vi "Compute Guess Fit Parameters.vi"(8 "error in (no error)":errorcluster, 9 "Additional Data":variant, 10 "Fit Model":T2, 11 "Data in":T3) -> (0 "error out":errorcluster, 1 "Additional LM Data":variant, 3 "Initial Fit Parameters":dbl[](array[numeric]), 4 "Parameter Bounds":T1={"parameter minimum"=[0.0, -inf, 0.0], "parameter maximum"=[inf, inf, inf]})   [LabVIEW 2019]
uses:
  Fit Models.ctl
  N Components Additional Fit Settings.ctl
  D-Only Fixed Parameters.ctl
  <vilib>/Utility/error.llb/DialogType.ctl
  <vilib>/Analysis/NI_AALPro.lvlib
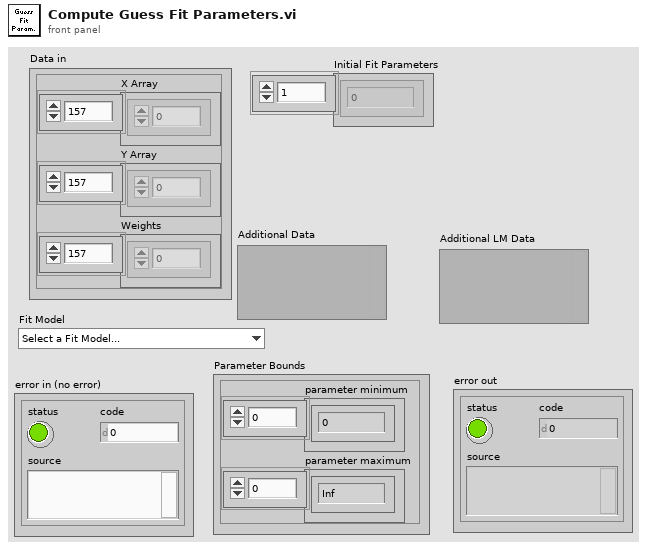
[diagram p1: front panel]
types:
  T1 = cluster{"parameter minimum":dbl[], "parameter maximum":dbl[]}
  T2 = typedef "Fit Models.ctl" = enum16{"Select a Fit Model...", "           Single Peak", "Gaussian", "Asymmetric Gaussian", "Lorentzian", "Asymmetric Lorentzian", "Gaussian/Lorentzian", "Lorentzian/Gaussian", "           Double Peak", "Two Gaussians", "Two Asymmetric Gaussians", "Two H-Connected Gaussians", "Two T-Connected Gaussians", "Two H-Connected Asymmetric Gaussians", "Two T-Connected Asymmetric Gaussians", "           Triple Peak", "Three Gaussians", "Three Asymmetric Gaussians", "              Decays", "Single Exponential", "Two Exponentials", "               ACF", "2D Gaussian ACF", "2D Gaussian + Blinking ACF", "2D Gaussian + Flow ACF", "3D Gaussian ACF", "3D Gaussian + Blinking ACF", "             Multiplot", "2D Gaussian ACF & 2D Gaussian + Flow ACF"}
  T3 = cluster{"X Array":dbl[], "Y Array":dbl[], "Weights":dbl[]}
  T4 = typedef "N Components Additional Fit Settings.ctl" = cluster{"Fixed Parameters":T5, "Cursor Coordinates":dbl[], "Data Split Point":i32}
  T5 = typedef "D-Only Fixed Parameters.ctl" = cluster{"Fix D-only Peak Location":bool, "Peak Location":dbl, "Fix D-only Peak FWHM":bool, "Peak FWHM":dbl}
  T6 = cluster{"initial amplitude":dbl, "initial center":dbl, "initial standard deviation":dbl, "offset":dbl}
  T7 = cluster{"amp min":dbl, "amp max":dbl, "damping min":dbl, "damping max":dbl, "offset min":dbl, "offset max":dbl}
  T8 = typedef "DialogType.ctl" = u16
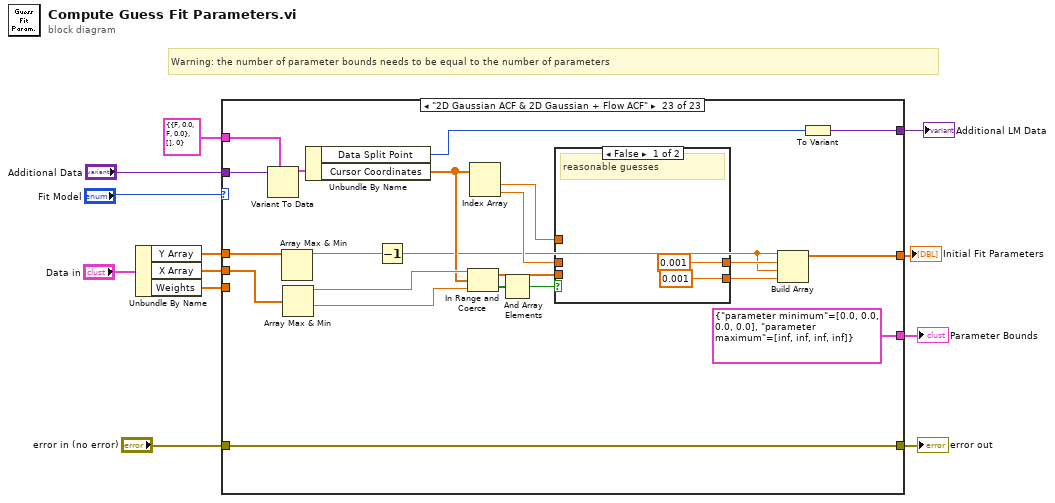
[diagram p0: block diagram]
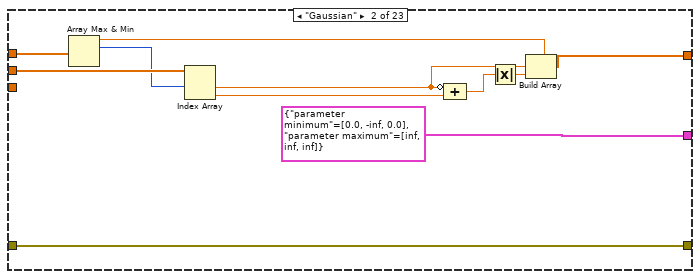
[diagram p3: hidden frame]
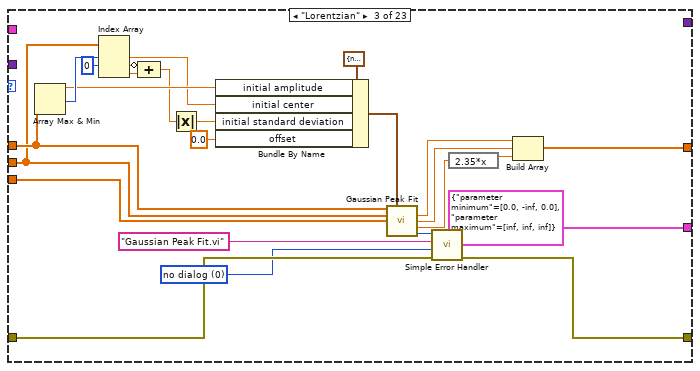
[diagram p4: hidden frame]
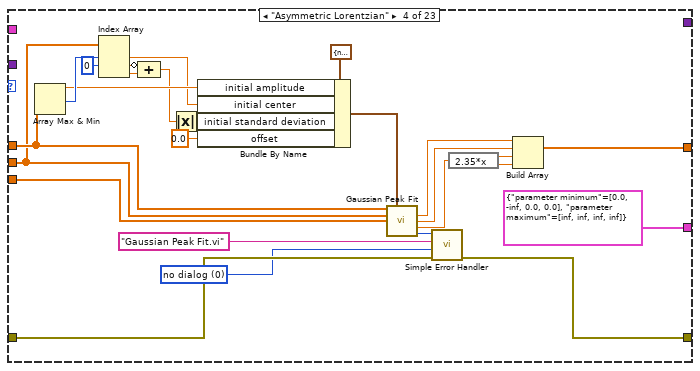
[diagram p5: hidden frame]
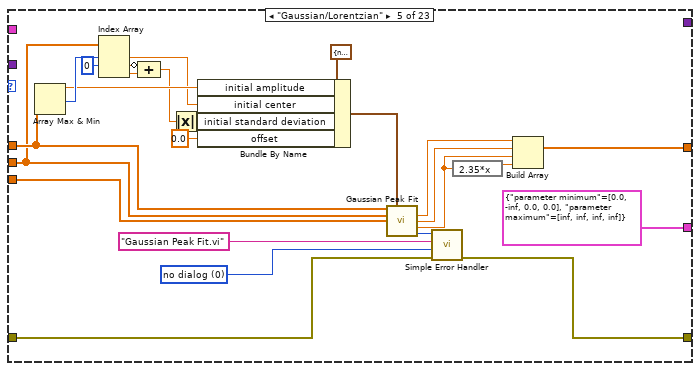
[diagram p6: hidden frame]
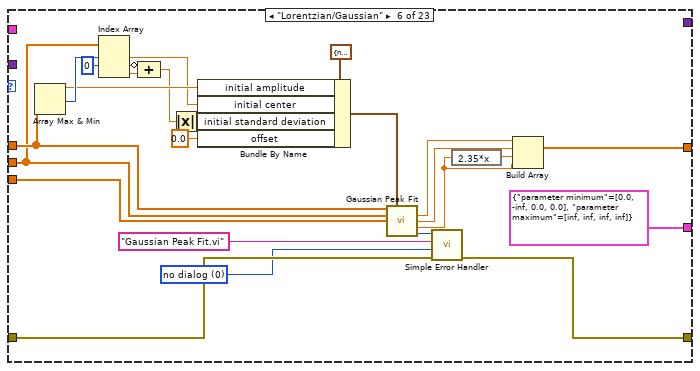
[diagram p7: hidden frame]
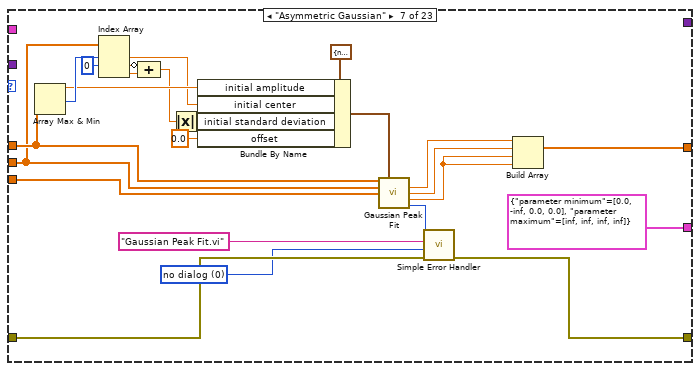
[diagram p8: hidden frame]
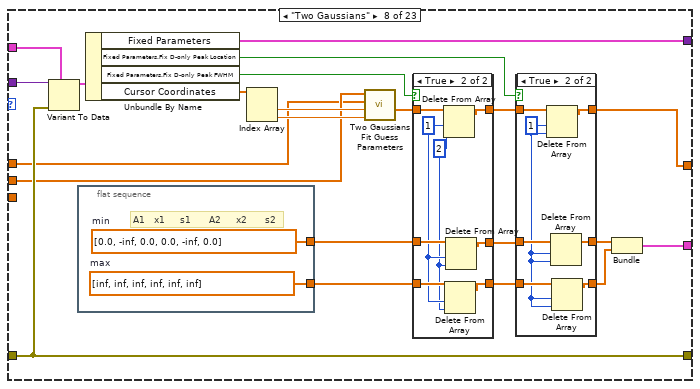
[diagram p9: hidden frame]
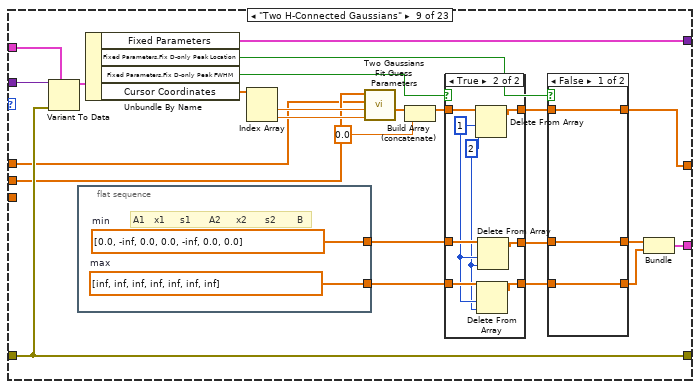
[diagram p12: hidden frame]
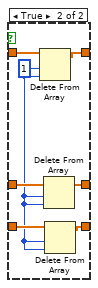
[diagram p14: hidden frame]
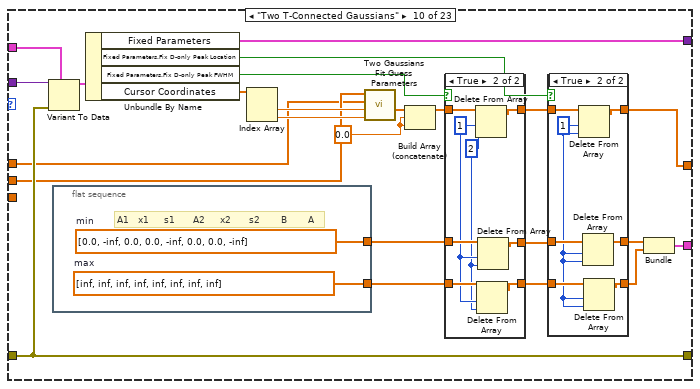
[diagram p15: hidden frame]
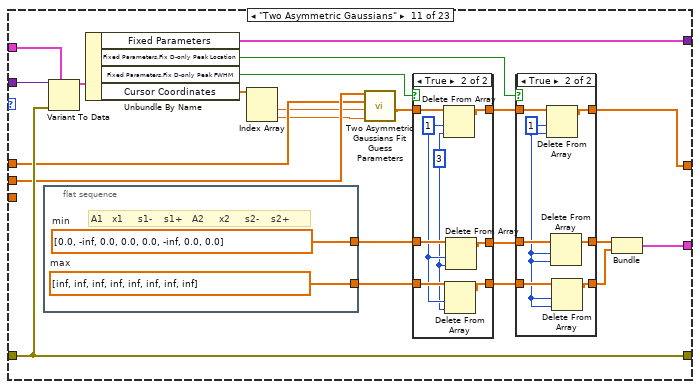
[diagram p18: hidden frame]
diagram:
  # "Warning: the number of parameter bounds needs to be equal to the number of parameters"
  n1 = Unbundle By Name("Data in") -> ("Y Array"=w8:dbl[], "X Array"=w7:dbl[], "Weights"=w6:dbl[])
  n2 = case shown="\"2D Gaussian ACF & 2D Gaussian + Flow ACF\"" "Fit Model" {
    tunnel: "error in (no error)" -> [w13 w24 w49 w74 w99 w124 w148 w169 w216 w263 w308 w355 w402 w446 w492 w523 w535 w552 w576 w601 w623 w648 w674]
    tunnel: [_ w15 w45 w71 w97 w122 w146 w154 w201 w248 w298 w335 w382 w437 w480 w518 w532 w549 w573 w598 w620 w645 w671] -> w11
    tunnel: [w13 w24 w43 w69 w95 w120 w144 w169 w216 w263 w308 w355 w402 w446 w492 w523 w535 w552 w576 w601 w623 w648 w674] -> w10
    tunnel: w8 -> [_ w22 w32 w58 w84 w109 w133 w163 w210 w257 w292 w339 w386 w431 w489 w526 w534 w551 w575 w600 w622 w647 w673]
    tunnel: w7 -> [_ w23 w31 w57 w83 w108 w132 w164 w211 w258 w293 w340 w387 w432 w490 w527 w533 w539 w564 w589 w609 w636 w663]
    tunnel: w6 -> [_ _ w39 w65 w91 w116 w140 _ _ _ _ _ _ _ _ w525 _ _ _ _ _ _ _]
    tunnel: [_ T1 {"parameter minimum"=[0.0, -inf, 0.0], "parameter maximum"=[inf, inf, inf]} ("Parameter Bounds") T1 {"parameter minimum"=[0.0, -inf, 0.0], "parameter maximum"=[inf, inf, inf]} ("Parameter Bounds") T1 {"parameter minimum"=[0.0, -inf, 0.0, 0.0], "parameter maximum"=[inf, inf, inf, inf]} ("Parameter Bounds") T1 {"parameter minimum"=[0.0, -inf, 0.0, 0.0], "parameter maximum"=[inf, inf, inf, inf]} ("Parameter Bounds") T1 {"parameter minimum"=[0.0, -inf, 0.0, 0.0], "parameter maximum"=[inf, inf, inf, inf]} ("Parameter Bounds") T1 {"parameter minimum"=[0.0, -inf, 0.0, 0.0], "parameter maximum"=[inf, inf, inf, inf]} ("Parameter Bounds") w151 w198 w245 w295 w342 w389 w434 w477 T1 {"parameter minimum"=[0.0, 0.0], "parameter maximum"=[inf, inf]} ("parameter bounds") T1 {"parameter minimum"=[0.0, 0.0, 0.0, 0.0], "parameter maximum"=[inf, inf, inf, inf]} ("parameter bounds") T1 {"parameter minimum"=[0.0, 0.0], "parameter maximum"=[inf, inf]} ("Parameter Bounds") T1 {"parameter minimum"=[0.0, 0.0, 0.0, 0.0], "parameter maximum"=[inf, inf, inf, inf]} ("Parameter Bounds") T1 {"parameter minimum"=[0.0, 0.0, 0.0], "parameter maximum"=[inf, inf, inf]} ("Parameter Bounds") T1 {"parameter minimum"=[0.0, 0.0, 0.0], "parameter maximum"=[inf, inf, inf]} ("Parameter Bounds") T1 {"parameter minimum"=[0.0, 0.0, 0.0, 0.0, 0.0], "parameter maximum"=[inf, inf, inf, inf, inf]} ("Parameter Bounds") T1 {"parameter minimum"=[0.0, 0.0, 0.0, 0.0], "parameter maximum"=[inf, inf, inf, inf]} ("Parameter Bounds")] -> w4
    tunnel: "Additional Data" -> [_ _ _ _ _ _ _ w170 w217 w264 w309 w356 w403 w447 w493 _ _ w547 w571 w596 w618 w643 w669]
    tunnel: [_ _ _ _ _ _ _ w150 w197 w244 w294 w341 w388 w433 w476 _ _ _ _ _ _ _ w653] -> w2
    tunnel: T4 {"Fixed Parameters"={"Fix D-only Peak Location"=FALSE, "Peak Location"=0.0, "Fix D-only Peak FWHM"=FALSE, "Peak FWHM"=0.0}, "Cursor Coordinates"=[], "Data Split Point"=0} ("N Components Additional Fit Settings") -> [_ _ _ _ _ _ _ w149 w194 w241 w288 w333 w380 w427 w473 _ _ w536 w555 w582 w606 w626 w657]
    frame "Select a Fit Model...", Default {
    }
    frame "Gaussian" {
      n3 = Array Max & Min(array=w22) -> (max value=w20:dbl, max index (indices)=w21:i32)  [unwired: 2 out]
      n4 = Index Array(array=w23, index #1=w21) -> (element #1=w19:dbl, element #2=w18:dbl)  [unwired: 1 in]
      n5 = Compound Arithmetic op=ADD(invert w19, w18) -> (w17:dbl)
      n6 = Absolute Value(x=w17) -> (abs(x)=w16:dbl)
      n7 = Build Array(w20, w19, w16) -> (w15:dbl[])
    }
    frame "Lorentzian" {
      w42 = T8 0 items=["no dialog", "OK message", "continue or stop message", "OK message + warnings", "continue/stop + warnings"] ("type of dialog (OK msg:1)")
      n8 = Array Max & Min(array=w32) -> (max value=w35:dbl, max index (indices)=w37:i32)  [unwired: 2 out]
      n9 = Index Array(array=w31, index #1=w37, index #2=0 ("index")) -> (element #1=w34:dbl, element #2=w29:dbl, element #3=w28:dbl)  [unwired: 1 in]
      n10 = Compound Arithmetic op=ADD(invert w29, w28) -> (w27:dbl)
      n11 = Absolute Value(x=w27) -> (abs(x)=w26:dbl)
      n12 = Bundle By Name(cluster=T6 {"initial amplitude"=nan, "initial center"=nan, "initial standard deviation"=nan, "offset"=nan} ("initial guess"), "initial amplitude"=w35, "initial center"=w34, "initial standard deviation"=w26, "offset"=0.0) -> (w25:T6)
      n13 = call <vilib>:"Gaussian Peak Fit.vi"("Y"=w32, "initial guess"=w25, "X"=w31, "Weight"=w39) -> ("amplitude"=w44:dbl, "center"=w46:dbl, "standard deviation"=w47:dbl, "error"=w41:i32)  [unwired: 5 in, 3 out]
      n14 = call <vilib>:"Simple Error Handler.vi"("error code (no error:0)"=w41, "error source (\" \")"="Gaussian Peak Fit.vi" ("error source (\" \")"), "type of dialog (OK msg:1)"=w42, "error in (no error)"=w49) -> ("error out"=w43:errorcluster)  [unwired: 1 in, 4 out]
      n15 = expression code="2.35*x"(w47) -> (w48:dbl)
      n16 = Build Array(w44, w46, w48) -> (w45:dbl[])
    }
    frame "Asymmetric Lorentzian" {
      w68 = T8 0 items=["no dialog", "OK message", "continue or stop message", "OK message + warnings", "continue/stop + warnings"] ("type of dialog (OK msg:1)")
      n17 = Array Max & Min(array=w58) -> (max value=w61:dbl, max index (indices)=w63:i32)  [unwired: 2 out]
      n18 = Index Array(array=w57, index #1=w63, index #2=0 ("index")) -> (element #1=w60:dbl, element #2=w55:dbl, element #3=w54:dbl)  [unwired: 1 in]
      n19 = Compound Arithmetic op=ADD(invert w55, w54) -> (w53:dbl)
      n20 = Absolute Value(x=w53) -> (abs(x)=w52:dbl)
      n21 = Bundle By Name(cluster=T6 {"initial amplitude"=nan, "initial center"=nan, "initial standard deviation"=nan, "offset"=nan} ("initial guess"), "initial amplitude"=w61, "initial center"=w60, "initial standard deviation"=w52, "offset"=0.0) -> (w51:T6)
      n22 = call <vilib>:"Gaussian Peak Fit.vi"("Y"=w58, "initial guess"=w51, "X"=w57, "Weight"=w65) -> ("amplitude"=w70:dbl, "center"=w72:dbl, "standard deviation"=w73:dbl, "error"=w67:i32)  [unwired: 5 in, 3 out]
      n23 = call <vilib>:"Simple Error Handler.vi"("error code (no error:0)"=w67, "error source (\" \")"="Gaussian Peak Fit.vi" ("error source (\" \")"), "type of dialog (OK msg:1)"=w68, "error in (no error)"=w74) -> ("error out"=w69:errorcluster)  [unwired: 1 in, 4 out]
      n24 = expression code="2.35*x"(w73) -> (w50:dbl)
      n25 = Build Array(w70, w72, w50, w50) -> (w71:dbl[])
    }
    frame "Gaussian/Lorentzian" {
      w94 = T8 0 items=["no dialog", "OK message", "continue or stop message", "OK message + warnings", "continue/stop + warnings"] ("type of dialog (OK msg:1)")
      n26 = Array Max & Min(array=w84) -> (max value=w87:dbl, max index (indices)=w89:i32)  [unwired: 2 out]
      n27 = Index Array(array=w83, index #1=w89, index #2=0 ("index")) -> (element #1=w86:dbl, element #2=w81:dbl, element #3=w80:dbl)  [unwired: 1 in]
      n28 = Compound Arithmetic op=ADD(invert w81, w80) -> (w79:dbl)
      n29 = Absolute Value(x=w79) -> (abs(x)=w78:dbl)
      n30 = Bundle By Name(cluster=T6 {"initial amplitude"=nan, "initial center"=nan, "initial standard deviation"=nan, "offset"=nan} ("initial guess"), "initial amplitude"=w87, "initial center"=w86, "initial standard deviation"=w78, "offset"=0.0) -> (w77:T6)
      n31 = call <vilib>:"Gaussian Peak Fit.vi"("Y"=w84, "initial guess"=w77, "X"=w83, "Weight"=w91) -> ("amplitude"=w96:dbl, "center"=w98:dbl, "standard deviation"=w75:dbl, "error"=w93:i32)  [unwired: 5 in, 3 out]
      n32 = call <vilib>:"Simple Error Handler.vi"("error code (no error:0)"=w93, "error source (\" \")"="Gaussian Peak Fit.vi" ("error source (\" \")"), "type of dialog (OK msg:1)"=w94, "error in (no error)"=w99) -> ("error out"=w95:errorcluster)  [unwired: 1 in, 4 out]
      n33 = expression code="2.35*x"(w75) -> (w76:dbl)
      n34 = Build Array(w96, w98, w75, w76) -> (w97:dbl[])
    }
    frame "Lorentzian/Gaussian" {
      w119 = T8 0 items=["no dialog", "OK message", "continue or stop message", "OK message + warnings", "continue/stop + warnings"] ("type of dialog (OK msg:1)")
      n35 = Array Max & Min(array=w109) -> (max value=w112:dbl, max index (indices)=w114:i32)  [unwired: 2 out]
      n36 = Index Array(array=w108, index #1=w114, index #2=0 ("index")) -> (element #1=w111:dbl, element #2=w106:dbl, element #3=w105:dbl)  [unwired: 1 in]
      n37 = Compound Arithmetic op=ADD(invert w106, w105) -> (w104:dbl)
      n38 = Absolute Value(x=w104) -> (abs(x)=w103:dbl)
      n39 = Bundle By Name(cluster=T6 {"initial amplitude"=nan, "initial center"=nan, "initial standard deviation"=nan, "offset"=nan} ("initial guess"), "initial amplitude"=w112, "initial center"=w111, "initial standard deviation"=w103, "offset"=0.0) -> (w102:T6)
      n40 = call <vilib>:"Gaussian Peak Fit.vi"("Y"=w109, "initial guess"=w102, "X"=w108, "Weight"=w116) -> ("amplitude"=w121:dbl, "center"=w123:dbl, "standard deviation"=w100:dbl, "error"=w118:i32)  [unwired: 5 in, 3 out]
      n41 = call <vilib>:"Simple Error Handler.vi"("error code (no error:0)"=w118, "error source (\" \")"="Gaussian Peak Fit.vi" ("error source (\" \")"), "type of dialog (OK msg:1)"=w119, "error in (no error)"=w124) -> ("error out"=w120:errorcluster)  [unwired: 1 in, 4 out]
      n42 = expression code="2.35*x"(w100) -> (w101:dbl)
      n43 = Build Array(w121, w123, w101, w100) -> (w122:dbl[])
    }
    frame "Asymmetric Gaussian" {
      w143 = T8 0 items=["no dialog", "OK message", "continue or stop message", "OK message + warnings", "continue/stop + warnings"] ("type of dialog (OK msg:1)")
      n44 = Array Max & Min(array=w133) -> (max value=w136:dbl, max index (indices)=w138:i32)  [unwired: 2 out]
      n45 = Index Array(array=w132, index #1=w138, index #2=0 ("index")) -> (element #1=w135:dbl, element #2=w130:dbl, element #3=w129:dbl)  [unwired: 1 in]
      n46 = Compound Arithmetic op=ADD(invert w130, w129) -> (w128:dbl)
      n47 = Absolute Value(x=w128) -> (abs(x)=w127:dbl)
      n48 = Bundle By Name(cluster=T6 {"initial amplitude"=nan, "initial center"=nan, "initial standard deviation"=nan, "offset"=nan} ("initial guess"), "initial amplitude"=w136, "initial center"=w135, "initial standard deviation"=w127, "offset"=0.0) -> (w126:T6)
      n49 = call <vilib>:"Gaussian Peak Fit.vi"("Y"=w133, "initial guess"=w126, "X"=w132, "Weight"=w140) -> ("amplitude"=w145:dbl, "center"=w147:dbl, "standard deviation"=w125:dbl, "error"=w142:i32)  [unwired: 5 in, 3 out]
      n50 = call <vilib>:"Simple Error Handler.vi"("error code (no error:0)"=w142, "error source (\" \")"="Gaussian Peak Fit.vi" ("error source (\" \")"), "type of dialog (OK msg:1)"=w143, "error in (no error)"=w148) -> ("error out"=w144:errorcluster)  [unwired: 1 in, 4 out]
      n51 = Build Array(w145, w147, w125, w125) -> (w146:dbl[])
    }
    frame "Two Gaussians" {
      n52 = Variant To Data(error in=w169, type=w149, Variant=w170) -> (data=w168:T4)  [unwired: 1 out]
      n53 = flat-sequence {
        tunnel: [w172] -> w161
        tunnel: [w171] -> w160
        frame #0 {
          w171 = dbl[] [inf, inf, inf, inf, inf, inf]  # max
          w172 = dbl[] [0.0, -inf, 0.0, 0.0, -inf, 0.0]  # min
          # "A1   x1     s1      A2     x2      s2"
        }
      }
      n54 = Unbundle By Name(w168) -> ("Fixed Parameters"=w150:T5, "Fixed Parameters.Fix D-only Peak Location"=w155:bool, "Fixed Parameters.Fix D-only Peak FWHM"=w156:bool, "Cursor Coordinates"=w167:dbl[])
      n55 = Index Array(array=w167) -> (element #1=w166:dbl, element #2=w165:dbl)  [unwired: 2 in]
      n56 = call "Two Gaussians Fit Guess Parameters.vi"("Cursor X 2"=w165, "Cursor X 1"=w166, "Y Array"=w163, "X Array"=w164) -> ("Guess Parameters Array"=w162:dbl[])  [unwired: 5 in, 2 out]
      n57 = case shown="True" w156 {
        tunnel: w162 -> [w175 w183]
        tunnel: [w175 w182] -> w157
        tunnel: w161 -> [w174 w181]
        tunnel: w160 -> [w173 w180]
        tunnel: [w173 w177] -> w159
        tunnel: [w174 w176] -> w158
        frame False {
        }
        frame True {
          w178 = 2 ("index")
          w179 = 1 ("length")
          n58 = Delete From Array(array=w183, length=w179, index=w178) -> (array with subset deleted=w182:dbl[])  [unwired: 1 out]
          n59 = Delete From Array(array=w180, length=w179, index=w178) -> (array with subset deleted=w177:dbl[])  [unwired: 1 out]
          n60 = Delete From Array(array=w181, length=w179, index=w178) -> (array with subset deleted=w176:dbl[])  [unwired: 1 out]
        }
      }
      n61 = case shown="True" w155 {
        tunnel: w157 -> [w186 w193]
        tunnel: [w186 w192] -> w154
        tunnel: w158 -> [w185 w191]
        tunnel: w159 -> [w184 w189]
        tunnel: [w185 w190] -> w153
        tunnel: [w184 w187] -> w152
        frame False {
        }
        frame True {
          w188 = 1 ("length")
          n62 = Delete From Array(array=w193, length=w188, index=w188) -> (array with subset deleted=w192:dbl[])  [unwired: 1 out]
          n63 = Delete From Array(array=w191, length=w188, index=w188) -> (array with subset deleted=w190:dbl[])  [unwired: 1 out]
          n64 = Delete From Array(array=w189, length=w188, index=w188) -> (array with subset deleted=w187:dbl[])  [unwired: 1 out]
        }
      }
      n65 = Bundle("min"=w153, "max"=w152) -> (w151:cluster{"min":dbl[], "max":dbl[]})  [unwired: 1 in]
    }
    frame "Two H-Connected Gaussians" {
      n66 = Variant To Data(error in=w216, type=w194, Variant=w217) -> (data=w215:T4)  [unwired: 1 out]
      n67 = flat-sequence {
        tunnel: [w219] -> w208
        tunnel: [w218] -> w207
        frame #0 {
          w218 = dbl[] [inf, inf, inf, inf, inf, inf, inf]  # max
          w219 = dbl[] [0.0, -inf, 0.0, 0.0, -inf, 0.0, 0.0]  # min
          # "A1   x1     s1      A2     x2      s2       B"
        }
      }
      n68 = Unbundle By Name(w215) -> ("Fixed Parameters"=w197:T5, "Fixed Parameters.Fix D-only Peak Location"=w202:bool, "Fixed Parameters.Fix D-only Peak FWHM"=w203:bool, "Cursor Coordinates"=w214:dbl[])
      n69 = Index Array(array=w214) -> (element #1=w213:dbl, element #2=w212:dbl)  [unwired: 2 in]
      n70 = call "Two Gaussians Fit Guess Parameters.vi"("Cursor X 2"=w212, "Cursor X 1"=w213, "Y Array"=w210, "X Array"=w211) -> ("Guess Parameters Array"=w209:dbl[])  [unwired: 5 in, 2 out]
      n71 = Build Array (concatenate)(w209, 0.0 ("Numeric")) -> (w196:dbl[])
      n72 = case shown="True" w203 {
        tunnel: w196 -> [w222 w230]
        tunnel: [w222 w229] -> w204
        tunnel: w208 -> [w221 w228]
        tunnel: w207 -> [w220 w227]
        tunnel: [w220 w224] -> w206
        tunnel: [w221 w223] -> w205
        frame False {
        }
        frame True {
          w225 = 2 ("index")
          w226 = 1 ("length")
          n73 = Delete From Array(array=w230, length=w226, index=w225) -> (array with subset deleted=w229:dbl[])  [unwired: 1 out]
          n74 = Delete From Array(array=w227, length=w226, index=w225) -> (array with subset deleted=w224:dbl[])  [unwired: 1 out]
          n75 = Delete From Array(array=w228, length=w226, index=w225) -> (array with subset deleted=w223:dbl[])  [unwired: 1 out]
        }
      }
      n76 = case shown="False" w202 {
        tunnel: w204 -> [w233 w240]
        tunnel: [w233 w239] -> w201
        tunnel: w205 -> [w232 w238]
        tunnel: w206 -> [w231 w236]
        tunnel: [w232 w237] -> w200
        tunnel: [w231 w234] -> w199
        frame False {
        }
        frame True {
          w235 = 1 ("length")
          n77 = Delete From Array(array=w240, length=w235, index=w235) -> (array with subset deleted=w239:dbl[])  [unwired: 1 out]
          n78 = Delete From Array(array=w238, length=w235, index=w235) -> (array with subset deleted=w237:dbl[])  [unwired: 1 out]
          n79 = Delete From Array(array=w236, length=w235, index=w235) -> (array with subset deleted=w234:dbl[])  [unwired: 1 out]
        }
      }
      n80 = Bundle("min"=w200, "max"=w199) -> (w198:cluster{"min":dbl[], "max":dbl[]})  [unwired: 1 in]
    }
    frame "Two T-Connected Gaussians" {
      w242 = 0.0 ("Numeric")
      n81 = Variant To Data(error in=w263, type=w241, Variant=w264) -> (data=w262:T4)  [unwired: 1 out]
      n82 = flat-sequence {
        tunnel: [w266] -> w255
        tunnel: [w265] -> w254
        frame #0 {
          w265 = dbl[] [inf, inf, inf, inf, inf, inf, inf, inf]  # max
          w266 = dbl[] [0.0, -inf, 0.0, 0.0, -inf, 0.0, 0.0, -inf]  # min
          # "A1   x1     s1      A2     x2      s2       B       A"
        }
      }
      n83 = Unbundle By Name(w262) -> ("Fixed Parameters"=w244:T5, "Fixed Parameters.Fix D-only Peak Location"=w249:bool, "Fixed Parameters.Fix D-only Peak FWHM"=w250:bool, "Cursor Coordinates"=w261:dbl[])
      n84 = Index Array(array=w261) -> (element #1=w260:dbl, element #2=w259:dbl)  [unwired: 2 in]
      n85 = call "Two Gaussians Fit Guess Parameters.vi"("Cursor X 2"=w259, "Cursor X 1"=w260, "Y Array"=w257, "X Array"=w258) -> ("Guess Parameters Array"=w256:dbl[])  [unwired: 5 in, 2 out]
      n86 = Build Array (concatenate)(w256, w242, w242) -> (w243:dbl[])
      n87 = case shown="True" w250 {
        tunnel: w243 -> [w269 w277]
        tunnel: [w269 w276] -> w251
        tunnel: w255 -> [w268 w275]
        tunnel: w254 -> [w267 w274]
        tunnel: [w267 w271] -> w253
        tunnel: [w268 w270] -> w252
        frame False {
        }
        frame True {
          w272 = 2 ("index")
          w273 = 1 ("length")
          n88 = Delete From Array(array=w277, length=w273, index=w272) -> (array with subset deleted=w276:dbl[])  [unwired: 1 out]
          n89 = Delete From Array(array=w274, length=w273, index=w272) -> (array with subset deleted=w271:dbl[])  [unwired: 1 out]
          n90 = Delete From Array(array=w275, length=w273, index=w272) -> (array with subset deleted=w270:dbl[])  [unwired: 1 out]
        }
      }
      n91 = case shown="True" w249 {
        tunnel: w251 -> [w280 w287]
        tunnel: [w280 w286] -> w248
        tunnel: w252 -> [w279 w285]
        tunnel: w253 -> [w278 w283]
        tunnel: [w279 w284] -> w247
        tunnel: [w278 w281] -> w246
        frame False {
        }
        frame True {
          w282 = 1 ("length")
          n92 = Delete From Array(array=w287, length=w282, index=w282) -> (array with subset deleted=w286:dbl[])  [unwired: 1 out]
          n93 = Delete From Array(array=w285, length=w282, index=w282) -> (array with subset deleted=w284:dbl[])  [unwired: 1 out]
          n94 = Delete From Array(array=w283, length=w282, index=w282) -> (array with subset deleted=w281:dbl[])  [unwired: 1 out]
        }
      }
      n95 = Bundle("min"=w247, "max"=w246) -> (w245:cluster{"min":dbl[], "max":dbl[]})  [unwired: 1 in]
    }
    frame "Two Asymmetric Gaussians" {
      n96 = flat-sequence {
        tunnel: [w311] -> w305
        tunnel: [w310] -> w304
        frame #0 {
          w310 = dbl[] [inf, inf, inf, inf, inf, inf, inf, inf]  # max
          w311 = dbl[] [0.0, -inf, 0.0, 0.0, 0.0, -inf, 0.0, 0.0]  # min
          # "A1   x1     s1-    s1+   A2     x2     s2-    s2+"
        }
      }
      n97 = Variant To Data(error in=w308, type=w288, Variant=w309) -> (data=w307:T4)  [unwired: 1 out]
      n98 = Unbundle By Name(w307) -> ("Fixed Parameters"=w294:T5, "Fixed Parameters.Fix D-only Peak Location"=w299:bool, "Fixed Parameters.Fix D-only Peak FWHM"=w300:bool, "Cursor Coordinates"=w306:dbl[])
      n99 = Index Array(array=w306) -> (element #1=w291:dbl, element #2=w290:dbl)  [unwired: 2 in]
      n100 = call "Two Asymmetric Gaussians Fit Guess Parameters.vi"("Cursor X 2"=w290, "Cursor X 1"=w291, "Y Array"=w292, "X Array"=w293) -> ("Guess Parameters Array"=w289:dbl[])  [unwired: 5 in, 2 out]
      n101 = case shown="True" w300 {
        tunnel: w289 -> [w314 w322]
        tunnel: [w314 w321] -> w301
        tunnel: w305 -> [w313 w320]
        tunnel: w304 -> [w312 w319]
        tunnel: [w312 w316] -> w303
        tunnel: [w313 w315] -> w302
        frame False {
        }
        frame True {
          w317 = 3 ("index")
          w318 = 1 ("length")
          n102 = Delete From Array(array=w322, length=w318, index=w317) -> (array with subset deleted=w321:dbl[])  [unwired: 1 out]
          n103 = Delete From Array(array=w319, length=w318, index=w317) -> (array with subset deleted=w316:dbl[])  [unwired: 1 out]
          n104 = Delete From Array(array=w320, length=w318, index=w317) -> (array with subset deleted=w315:dbl[])  [unwired: 1 out]
        }
      }
      n105 = case shown="True" w299 {
        tunnel: w301 -> [w325 w332]
        tunnel: [w325 w331] -> w298
        tunnel: w302 -> [w324 w330]
        tunnel: w303 -> [w323 w328]
        tunnel: [w324 w329] -> w297
        tunnel: [w323 w326] -> w296
        frame False {
        }
        frame True {
          w327 = 1 ("length")
          n106 = Delete From Array(array=w332, length=w327, index=w327) -> (array with subset deleted=w331:dbl[])  [unwired: 1 out]
          n107 = Delete From Array(array=w330, length=w327, index=w327) -> (array with subset deleted=w329:dbl[])  [unwired: 1 out]
          n108 = Delete From Array(array=w328, length=w327, index=w327) -> (array with subset deleted=w326:dbl[])  [unwired: 1 out]
        }
      }
      n109 = Bundle("min"=w297, "max"=w296) -> (w295:cluster{"min":dbl[], "max":dbl[]})  [unwired: 1 in]
    }
    frame "Two H-Connected Asymmetric Gaussians" {
      n110 = flat-sequence {
        tunnel: [w358] -> w352
        tunnel: [w357] -> w351
        frame #0 {
          w357 = dbl[] [inf, inf, inf, inf, inf, inf, inf, inf, inf]  # max
          w358 = dbl[] [0.0, -inf, 0.0, 0.0, 0.0, -inf, 0.0, 0.0, 0.0]  # min
          # "A1   x1     s1-    s1+   A2     x2     s2-    s2+     B"
        }
      }
      n111 = Variant To Data(error in=w355, type=w333, Variant=w356) -> (data=w354:T4)  [unwired: 1 out]
      n112 = Unbundle By Name(w354) -> ("Fixed Parameters"=w341:T5, "Fixed Parameters.Fix D-only Peak Location"=w346:bool, "Fixed Parameters.Fix D-only Peak FWHM"=w347:bool, "Cursor Coordinates"=w353:dbl[])
      n113 = Index Array(array=w353) -> (element #1=w338:dbl, element #2=w337:dbl)  [unwired: 2 in]
      n114 = call "Two Asymmetric Gaussians Fit Guess Parameters.vi"("Cursor X 2"=w337, "Cursor X 1"=w338, "Y Array"=w339, "X Array"=w340) -> ("Guess Parameters Array"=w336:dbl[])  [unwired: 5 in, 2 out]
      n115 = case shown="True" w347 {
        tunnel: w336 -> [w361 w369]
        tunnel: [w361 w368] -> w348
        tunnel: w352 -> [w360 w367]
        tunnel: w351 -> [w359 w366]
        tunnel: [w359 w363] -> w350
        tunnel: [w360 w362] -> w349
        frame False {
        }
        frame True {
          w364 = 3 ("index")
          w365 = 1 ("length")
          n116 = Delete From Array(array=w369, length=w365, index=w364) -> (array with subset deleted=w368:dbl[])  [unwired: 1 out]
          n117 = Delete From Array(array=w366, length=w365, index=w364) -> (array with subset deleted=w363:dbl[])  [unwired: 1 out]
          n118 = Delete From Array(array=w367, length=w365, index=w364) -> (array with subset deleted=w362:dbl[])  [unwired: 1 out]
        }
      }
      n119 = case shown="True" w346 {
        tunnel: w348 -> [w372 w379]
        tunnel: [w372 w378] -> w345
        tunnel: w349 -> [w371 w377]
        tunnel: w350 -> [w370 w375]
        tunnel: [w371 w376] -> w344
        tunnel: [w370 w373] -> w343
        frame False {
        }
        frame True {
          w374 = 1 ("length")
          n120 = Delete From Array(array=w379, length=w374, index=w374) -> (array with subset deleted=w378:dbl[])  [unwired: 1 out]
          n121 = Delete From Array(array=w377, length=w374, index=w374) -> (array with subset deleted=w376:dbl[])  [unwired: 1 out]
          n122 = Delete From Array(array=w375, length=w374, index=w374) -> (array with subset deleted=w373:dbl[])  [unwired: 1 out]
        }
      }
      n123 = Bundle("min"=w344, "max"=w343) -> (w342:cluster{"min":dbl[], "max":dbl[]})  [unwired: 1 in]
      n124 = Build Array (concatenate)(w345, 0.0 ("Numeric")) -> (w335:dbl[])
    }
    frame "Two T-Connected Asymmetric Gaussians" {
      w381 = 0.0 ("Numeric")
      n125 = flat-sequence {
        tunnel: [w405] -> w399
        tunnel: [w404] -> w398
        frame #0 {
          w404 = dbl[] [inf, inf, inf, inf, inf, inf, inf, inf, inf, inf]  # max
          w405 = dbl[] [0.0, -inf, 0.0, 0.0, 0.0, -inf, 0.0, 0.0, 0.0, -inf]  # min
          # "A1   x1     s1-    s1+   A2     x2     s2-    s2+     B      A"
        }
      }
      n126 = Variant To Data(error in=w402, type=w380, Variant=w403) -> (data=w401:T4)  [unwired: 1 out]
      n127 = Unbundle By Name(w401) -> ("Fixed Parameters"=w388:T5, "Fixed Parameters.Fix D-only Peak Location"=w393:bool, "Fixed Parameters.Fix D-only Peak FWHM"=w394:bool, "Cursor Coordinates"=w400:dbl[])
      n128 = Index Array(array=w400) -> (element #1=w385:dbl, element #2=w384:dbl)  [unwired: 2 in]
      n129 = call "Two Asymmetric Gaussians Fit Guess Parameters.vi"("Cursor X 2"=w384, "Cursor X 1"=w385, "Y Array"=w386, "X Array"=w387) -> ("Guess Parameters Array"=w383:dbl[])  [unwired: 5 in, 2 out]
      n130 = case shown="True" w394 {
        tunnel: w383 -> [w408 w416]
        tunnel: [w408 w415] -> w395
        tunnel: w399 -> [w407 w414]
        tunnel: w398 -> [w406 w413]
        tunnel: [w406 w410] -> w397
        tunnel: [w407 w409] -> w396
        frame False {
        }
        frame True {
          w411 = 3 ("index")
          w412 = 1 ("length")
          n131 = Delete From Array(array=w416, length=w412, index=w411) -> (array with subset deleted=w415:dbl[])  [unwired: 1 out]
          n132 = Delete From Array(array=w413, length=w412, index=w411) -> (array with subset deleted=w410:dbl[])  [unwired: 1 out]
          n133 = Delete From Array(array=w414, length=w412, index=w411) -> (array with subset deleted=w409:dbl[])  [unwired: 1 out]
        }
      }
      n134 = case shown="True" w393 {
        tunnel: w395 -> [w419 w426]
        tunnel: [w419 w425] -> w392
        tunnel: w396 -> [w418 w424]
        tunnel: w397 -> [w417 w422]
        tunnel: [w418 w423] -> w391
        tunnel: [w417 w420] -> w390
        frame False {
        }
        frame True {
          w421 = 1 ("length")
          n135 = Delete From Array(array=w426, length=w421, index=w421) -> (array with subset deleted=w425:dbl[])  [unwired: 1 out]
          n136 = Delete From Array(array=w424, length=w421, index=w421) -> (array with subset deleted=w423:dbl[])  [unwired: 1 out]
          n137 = Delete From Array(array=w422, length=w421, index=w421) -> (array with subset deleted=w420:dbl[])  [unwired: 1 out]
        }
      }
      n138 = Bundle("min"=w391, "max"=w390) -> (w389:cluster{"min":dbl[], "max":dbl[]})  [unwired: 1 in]
      n139 = Build Array (concatenate)(w392, w381, w381) -> (w382:dbl[])
    }
    frame "Three Asymmetric Gaussians" {
      n140 = flat-sequence {
        tunnel: [w451] -> w444
        tunnel: [w449] -> w443
        frame #0 {
          w448 = dbl[] [inf, inf, inf, inf]  # max
          w450 = dbl[] [0.0, -inf, 0.0, 0.0]  # min
          # "A1   x1     s1-    s1+"
          n141 = Build Array (concatenate)(w450, w450, w450) -> (w451:dbl[])
          n142 = Build Array (concatenate)(w448, w448, w448) -> (w449:dbl[])
        }
      }
      n143 = Variant To Data(error in=w446, type=w427, Variant=w447) -> (data=w445:T4)  [unwired: 1 out]
      n144 = Unbundle By Name(w445) -> ("Fixed Parameters"=w433:T5, "Fixed Parameters.Fix D-only Peak Location"=w438:bool, "Fixed Parameters.Fix D-only Peak FWHM"=w439:bool, "Cursor Coordinates"=w430:dbl[])
      n145 = call "N Asymmetric Gaussians Fit Guess Parameters.vi"("N"=3, "Cursor X Array"=w430, "Y Array"=w431, "X Array"=w432) -> ("Guess Parameters Array"=w429:dbl[])  [unwired: 5 in, 2 out]
      n146 = case shown="True" w439 {
        tunnel: w429 -> [w454 w462]
        tunnel: [w454 w461] -> w440
        tunnel: w444 -> [w453 w460]
        tunnel: w443 -> [w452 w459]
        tunnel: [w452 w456] -> w442
        tunnel: [w453 w455] -> w441
        frame False {
        }
        frame True {
          w457 = 3 ("index")
          w458 = 1 ("length")
          n147 = Delete From Array(array=w462, length=w458, index=w457) -> (array with subset deleted=w461:dbl[])  [unwired: 1 out]
          n148 = Delete From Array(array=w459, length=w458, index=w457) -> (array with subset deleted=w456:dbl[])  [unwired: 1 out]
          n149 = Delete From Array(array=w460, length=w458, index=w457) -> (array with subset deleted=w455:dbl[])  [unwired: 1 out]
        }
      }
      n150 = case shown="True" w438 {
        tunnel: w440 -> [w465 w472]
        tunnel: [w465 w471] -> w437
        tunnel: w441 -> [w464 w470]
        tunnel: w442 -> [w463 w468]
        tunnel: [w464 w469] -> w436
        tunnel: [w463 w466] -> w435
        frame False {
        }
        frame True {
          w467 = 1 ("length")
          n151 = Delete From Array(array=w472, length=w467, index=w467) -> (array with subset deleted=w471:dbl[])  [unwired: 1 out]
          n152 = Delete From Array(array=w470, length=w467, index=w467) -> (array with subset deleted=w469:dbl[])  [unwired: 1 out]
          n153 = Delete From Array(array=w468, length=w467, index=w467) -> (array with subset deleted=w466:dbl[])  [unwired: 1 out]
        }
      }
      n154 = Bundle(w436, w435) -> (w434:cluster{dbl[], dbl[]})  [unwired: 1 in]
    }
    frame "Three Gaussians" {
      n155 = Variant To Data(error in=w492, type=w473, Variant=w493) -> (data=w491:T4)  [unwired: 1 out]
      n156 = flat-sequence {
        tunnel: [w495] -> w487
        tunnel: [w494] -> w486
        frame #0 {
          w494 = dbl[] [inf, inf, inf, inf, inf, inf, inf, inf, inf]  # max
          w495 = dbl[] [0.0, -inf, 0.0, 0.0, -inf, 0.0, 0.0, -inf, 0.0]  # min
          # "A1   x1     s1      A2     x2      s2       A3     x3      s3"
        }
      }
      n157 = Unbundle By Name(w491) -> ("Fixed Parameters"=w476:T5, "Fixed Parameters.Fix D-only Peak Location"=w481:bool, "Fixed Parameters.Fix D-only Peak FWHM"=w482:bool, "Cursor Coordinates"=w475:dbl[])
      n158 = call "N Gaussians Fit Guess Parameters.vi"("N"=3, "Cursor X Array"=w475, "Y Array"=w489, "X Array"=w490) -> ("Guess Parameters Array"=w488:dbl[])  [unwired: 5 in, 2 out]
      n159 = case shown="True" w482 {
        tunnel: w488 -> [w498 w506]
        tunnel: [w498 w505] -> w483
        tunnel: w487 -> [w497 w504]
        tunnel: w486 -> [w496 w503]
        tunnel: [w496 w500] -> w485
        tunnel: [w497 w499] -> w484
        frame False {
        }
        frame True {
          w501 = 2 ("index")
          w502 = 1 ("length")
          n160 = Delete From Array(array=w506, length=w502, index=w501) -> (array with subset deleted=w505:dbl[])  [unwired: 1 out]
          n161 = Delete From Array(array=w503, length=w502, index=w501) -> (array with subset deleted=w500:dbl[])  [unwired: 1 out]
          n162 = Delete From Array(array=w504, length=w502, index=w501) -> (array with subset deleted=w499:dbl[])  [unwired: 1 out]
        }
      }
      n163 = case shown="True" w481 {
        tunnel: w483 -> [w509 w516]
        tunnel: [w509 w515] -> w480
        tunnel: w484 -> [w508 w514]
        tunnel: w485 -> [w507 w512]
        tunnel: [w508 w513] -> w479
        tunnel: [w507 w510] -> w478
        frame False {
        }
        frame True {
          w511 = 1 ("length")
          n164 = Delete From Array(array=w516, length=w511, index=w511) -> (array with subset deleted=w515:dbl[])  [unwired: 1 out]
          n165 = Delete From Array(array=w514, length=w511, index=w511) -> (array with subset deleted=w513:dbl[])  [unwired: 1 out]
          n166 = Delete From Array(array=w512, length=w511, index=w511) -> (array with subset deleted=w510:dbl[])  [unwired: 1 out]
        }
      }
      n167 = Bundle("min"=w479, "max"=w478) -> (w477:cluster{"min":dbl[], "max":dbl[]})  [unwired: 1 in]
    }
    frame "Single Exponential" {
      w522 = T8 0 items=["no dialog", "OK message", "continue or stop message", "OK message + warnings", "continue/stop + warnings"] ("type of dialog (OK msg:1)")
      n168 = call <vilib>:"Exponential Fit.vi"("Y"=w526, "X"=w527, "Weight"=w525, "tolerance"=1e-08, "parameter bounds"=T7 {"amp min"=0.0, "amp max"=inf, "damping min"=-inf, "damping max"=0.0, "offset min"=0.0, "offset max"=0.0}) -> ("amplitude"=w521:dbl, "damping"=w520:dbl, "error"=w530:i32)  [unwired: 5 in, 3 out]
      n169 = call <vilib>:"Simple Error Handler.vi"("error code (no error:0)"=w530, "error source (\" \")"="Exponential Fit.vi" ("error source (\" \")"), "type of dialog (OK msg:1)"=w522, "error in (no error)"=w523) -> ()  [unwired: 1 in, 5 out]
      n170 = expression code="-1/x"(w520) -> (w519:dbl)
      n171 = Build Array(w521, w519) -> (w518:dbl[])
    }
    frame "Two Exponentials" {
      n172 = call "Double Exponential Guess Parameters.vi"("Y"=w534, "X"=w533) -> ("2-Exp Guess Parameters"=w532:dbl[])  [unwired: 9 in]
    }
    frame "2D Gaussian ACF" {
      n173 = Variant To Data(type=w536, Variant=w547) -> (data=w546:T4)  [unwired: 1 in, 1 out]
      n174 = Array Max & Min(array=w551) -> (max value=w550:dbl)  [unwired: 3 out]
      n175 = Array Max & Min(array=w539) -> (max value=w544:dbl, min value=w543:dbl)  [unwired: 2 out]
      n176 = Unbundle By Name(w546) -> ("Cursor Coordinates"=w545:dbl[])
      n177 = Index Array(array=w545) -> (element=w537:dbl)  [unwired: 1 in]
      n178 = Decrement(x=w550) -> (x-1=w538:dbl)
      n179 = In Range and Coerce(upper limit=w544, x=w537, lower limit=w543) -> (coerced(x)=w541:dbl, In Range?=w542:bool)
      n180 = case shown="True" w542 {
        tunnel: w541 -> [_ w554]
        tunnel: [0.001 ("Cursor.Cursor X") w554] -> w540
        frame False {
        }
        frame True {
          # "if cursor OK\nuse it as tau_D"
        }
      }
      n181 = Build Array(w538, w540) -> (w549:dbl[])
    }
    frame "2D Gaussian + Blinking ACF" {
      n182 = Variant To Data(type=w555, Variant=w571) -> (data=w570:T4)  [unwired: 1 in, 1 out]
      n183 = Array Max & Min(array=w575) -> (max value=w574:dbl)  [unwired: 3 out]
      n184 = Array Max & Min(array=w564) -> (max value=w568:dbl, min value=w567:dbl)  [unwired: 2 out]
      n185 = Unbundle By Name(w570) -> ("Cursor Coordinates"=w569:dbl[])
      n186 = Decrement(x=w574) -> (x-1=w556:dbl)
      n187 = Sort 1D Array(array=w569) -> (sorted array=w563:dbl[])
      n188 = In Range and Coerce(upper limit=w568, x=w563, lower limit=w567) -> (coerced(x)=w565:dbl[], In Range?=w566:bool[])
      n189 = Index Array(array=w563) -> (element #1=w557:dbl, element #2=w559:dbl)  [unwired: 2 in]
      n190 = And Array Elements(Boolean array=w566) -> (logical AND=w562:bool)
      n191 = case shown="True" w562 {
        tunnel: w565 -> [_ _]
        tunnel: [0.001 ("Cursor.Cursor X") w580] -> w560
        tunnel: w559 -> [_ w580]
        tunnel: [1e-06 ("Cursor.Cursor X") w579] -> w558
        tunnel: w557 -> [_ w579]
        frame False {
          # "reasonable guesses"
        }
        frame True {
          # "if cursors are OK\nuse them as tau_D > tau_B"
        }
      }
      n192 = Build Array(w556, w560, 0.1 ("max value"), w558) -> (w573:dbl[])
    }
    frame "2D Gaussian + Flow ACF" {
      n193 = Variant To Data(type=w582, Variant=w596) -> (data=w595:T4)  [unwired: 1 in, 1 out]
      n194 = Array Max & Min(array=w600) -> (max value=w599:dbl)  [unwired: 3 out]
      n195 = Array Max & Min(array=w589) -> (max value=w593:dbl, min value=w592:dbl)  [unwired: 2 out]
      n196 = Unbundle By Name(w595) -> ("Cursor Coordinates"=w594:dbl[])
      n197 = Decrement(x=w599) -> (x-1=w581:dbl)
      n198 = Sort 1D Array(array=w594) -> (sorted array=w588:dbl[])
      n199 = In Range and Coerce(upper limit=w593, x=w588, lower limit=w592) -> (coerced(x)=w590:dbl[], In Range?=w591:bool[])
      n200 = Index Array(array=w588) -> (element #1=w583:dbl, element #2=w585:dbl)  [unwired: 2 in]
      n201 = And Array Elements(Boolean array=w591) -> (logical AND=w587:bool)
      n202 = case shown="True" w587 {
        tunnel: w590 -> [_ _]
        tunnel: [0.001 ("Cursor.Cursor X") w605] -> w586
        tunnel: w585 -> [_ w604]
        tunnel: [0.001 ("Cursor.Cursor X") w604] -> w584
        tunnel: w583 -> [_ w605]
        frame False {
          # "reasonable guesses"
        }
        frame True {
          # "if cursors are OK\nuse them"
        }
      }
      n203 = Build Array(w581, w586, w584) -> (w598:dbl[])
    }
    frame "3D Gaussian ACF" {
      n204 = Variant To Data(type=w606, Variant=w618) -> (data=w617:T4)  [unwired: 1 in, 1 out]
      n205 = Array Max & Min(array=w622) -> (max value=w621:dbl)  [unwired: 3 out]
      n206 = Array Max & Min(array=w609) -> (max value=w614:dbl, min value=w613:dbl)  [unwired: 2 out]
      n207 = Unbundle By Name(w617) -> ("Cursor Coordinates"=w616:dbl[])
      n208 = Index Array(array=w616) -> (element=w615:dbl)  [unwired: 1 in]
      n209 = Decrement(x=w621) -> (x-1=w607:dbl)
      n210 = In Range and Coerce(upper limit=w614, x=w615, lower limit=w613) -> (coerced(x)=w611:dbl, In Range?=w612:bool)
      n211 = case shown="False" w612 {
        tunnel: w611 -> [_ w625]
        tunnel: [0.001 ("Cursor.Cursor X") w625] -> w610
        frame False {
        }
        frame True {
          # "if cursor OK\nuse it as tau_D"
        }
      }
      n212 = Build Array(w607, w610, 4.0 ("element")) -> (w620:dbl[])
    }
    frame "3D Gaussian + Blinking ACF" {
      n213 = Variant To Data(type=w626, Variant=w643) -> (data=w642:T4)  [unwired: 1 in, 1 out]
      n214 = Array Max & Min(array=w647) -> (max value=w646:dbl)  [unwired: 3 out]
      n215 = Array Max & Min(array=w636) -> (max value=w640:dbl, min value=w639:dbl)  [unwired: 2 out]
      n216 = Unbundle By Name(w642) -> ("Cursor Coordinates"=w641:dbl[])
      n217 = Decrement(x=w646) -> (x-1=w628:dbl)
      n218 = Sort 1D Array(array=w641) -> (sorted array=w635:dbl[])
      n219 = In Range and Coerce(upper limit=w640, x=w635, lower limit=w639) -> (coerced(x)=w637:dbl[], In Range?=w638:bool[])
      n220 = Index Array(array=w635) -> (element #1=w629:dbl, element #2=w631:dbl)  [unwired: 2 in]
      n221 = And Array Elements(Boolean array=w638) -> (logical AND=w634:bool)
      n222 = case shown="True" w634 {
        tunnel: w637 -> [_ _]
        tunnel: [0.001 ("Cursor.Cursor X") w652] -> w632
        tunnel: w631 -> [_ w652]
        tunnel: [1e-06 ("Cursor.Cursor X") w651] -> w630
        tunnel: w629 -> [_ w651]
        frame False {
          # "reasonable guesses"
        }
        frame True {
          # "if cursors are OK\nuse them as tau_D > tau_B"
        }
      }
      n223 = Build Array(w628, w632, 4.0 ("max value"), 0.1 ("max value"), w630) -> (w645:dbl[])
    }
    frame "2D Gaussian ACF & 2D Gaussian + Flow ACF" {
      n224 = Variant To Data(type=w657, Variant=w669) -> (data=w668:T4)  [unwired: 1 in, 1 out]
      n225 = Array Max & Min(array=w673) -> (max value=w672:dbl)  [unwired: 3 out]
      n226 = Array Max & Min(array=w663) -> (max value=w667:dbl, min value=w666:dbl)  [unwired: 2 out]
      n227 = Unbundle By Name(w668) -> ("Data Split Point"=w654:i32, "Cursor Coordinates"=w656:dbl[])
      n228 = Decrement(x=w672) -> (x-1=w655:dbl)
      n229 = In Range and Coerce(upper limit=w667, x=w656, lower limit=w666) -> (coerced(x)=w664:dbl[], In Range?=w665:bool[])
      n230 = Index Array(array=w656) -> (element #1=w658:dbl, element #2=w660:dbl)  [unwired: 2 in]
      n231 = And Array Elements(Boolean array=w665) -> (logical AND=w662:bool)
      n232 = case shown="False" w662 {
        tunnel: w664 -> [_ _]
        tunnel: [0.001 ("Cursor.Cursor X") w678] -> w661
        tunnel: w660 -> [_ w677]
        tunnel: [0.001 ("Cursor.Cursor X") w677] -> w659
        tunnel: w658 -> [_ w678]
        frame False {
          # "reasonable guesses"
        }
        frame True {
          # "if cursors are OK\nuse them"
        }
      }
      n233 = Build Array(w655, w661, w655, w659) -> (w671:dbl[])
      n234 = To Variant(anything=w654) -> (Variant=w653:variant)
    }
  }
  "Initial Fit Parameters" <- w11
  "error out" <- w10
  "Parameter Bounds" <- w4
  "Additional LM Data" <- w2
